vi "BuildCountertask.vi"(9 "Input Cluster":T2, 10 "Sample rate":dbl, 11 "Task cluster in":T1) -> (2 "CO.Pulse.Term":tag, 3 "Task cluster out":T1)   [LabVIEW 2018]
uses:
  Tasks_RT.ctl
  <vilib>/DAQmx/create/channels.llb/DAQmx Create Channel (CO-Pulse Generation-Frequency).vi
  <vilib>/DAQmx/configure/timing.llb/DAQmx Timing (Implicit).vi
  <vilib>/DAQmx/configure/trigger.llb/DAQmx Start Trigger (Digital Edge).vi
  <resource>/objmgr/daqmx.rc
panel:
  # "Tasks and errors"
  # "Tasks and errors"
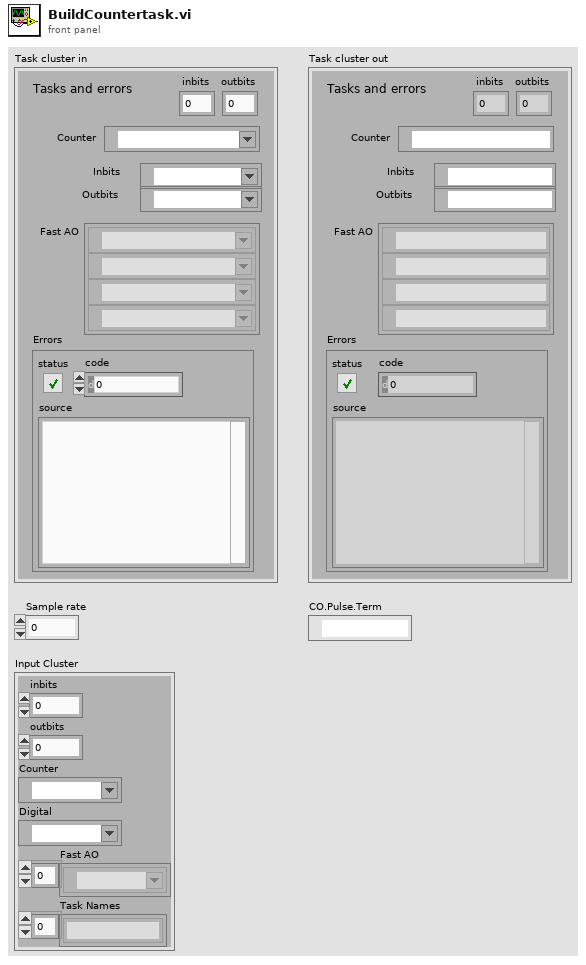
[diagram p1: front panel]
types:
  T1 = typedef "Tasks_RT.ctl" = cluster{"inbits":i32, "outbits":i32, "Counter":refnum<k21>, "Inbits":refnum<k21>, "Outbits":refnum<k21>, "Fast AO":refnum<k21>[], "Errors":errorcluster}
  T2 = cluster{"inbits":i32, "outbits":i32, "Counter":tag, "Digital":tag, "Fast AO":tag[], "Task Names":string[]}
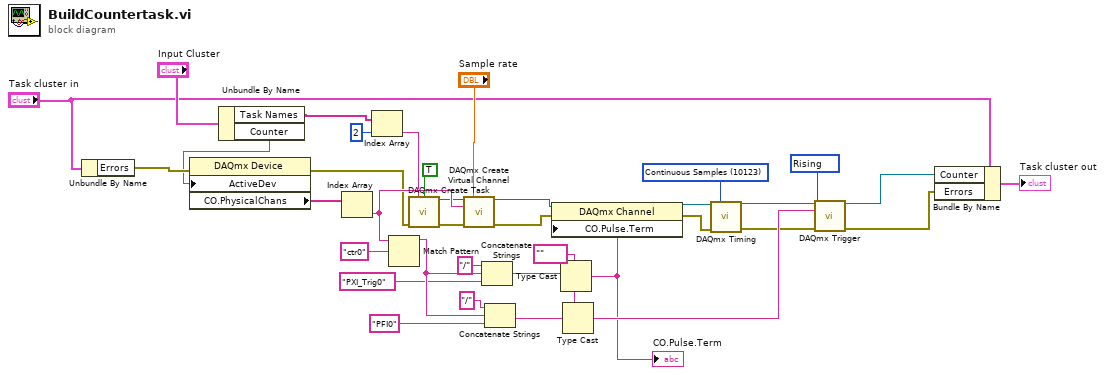
[diagram p0: block diagram]
diagram:
  w1 = 10280 items=["Rising"=10280, "Falling"=10171] ("edge")
  w22 = 10123 items=["Finite Samples"=10178, "Continuous Samples"=10123, "Hardware Timed Single Point"=12522] ("sample mode")
  w33 = tag "" ("CO.Pulse.Term")
  n1 = Unbundle By Name("Task cluster in") -> ("Errors"=w36:errorcluster)
  n2 = Unbundle By Name("Input Cluster") -> ("Task Names"=w13:string[], "Counter"=w4:tag)
  n3 = property class="DAQmx Device"(error in=w36, "ActiveDev"=w4) -> (error out=w15:errorcluster, "CO.PhysicalChans"=w14:tag[])  [unwired: 1 in, 1 out]
  n4 = Index Array(array=w14) -> (element=w16:tag)  [unwired: 1 in]
  n5 = Index Array(array=w13, index=2) -> (element=w12:string)
  n6 = Match Pattern(string=w16, regular expression="ctr0") -> (before substring=w29:string)  [unwired: 1 in, 3 out]
  n7 = call <vilib>:"DAQmx Create Task.vi"("new task name"=w12, "auto cleanup"=TRUE, "error in"=w15) -> ("task out"=w8:refnum<k21>, "error out"=w7:errorcluster)  [unwired: 11 in]
  n8 = call-poly <vilib>:"DAQmx Create Virtual Channel.vi"("task in"=w8, "frequency"="Sample rate", "counter"=w16, "error in"=w7) -> ("task out"=w5:refnum<k21>, "error out"=w6:errorcluster)  [unwired: 10 in]
  n9 = Concatenate Strings("/" ("string"), w29, "PXI_Trig0" ("string")) -> (w28:string)
  n10 = Concatenate Strings("/" ("string"), w29, "PFI0" ("string")) -> (w32:string)
  n11 = Type Cast(type=w33, x=w28) -> (*(type *) &x=w31:tag)
  "CO.Pulse.Term" <- w31
  n12 = property class="DAQmx Channel"(reference=w5, error in=w6, "CO.Pulse.Term"=w31) -> (reference out=w20:refnum<k21>, error out=w21:errorcluster)
  n13 = Type Cast(type=w33, x=w32) -> (*(type *) &x=w34:tag)
  n14 = call-poly <vilib>:"DAQmx Timing.vi"("task/channels in"=w20, "sample mode"=w22, "error in"=w21) -> ("task out"=w25:refnum<k21>, "error out"=w24:errorcluster)  [unwired: 11 in]
  n15 = call-poly <vilib>:"DAQmx Trigger.vi"("task/channels in"=w25, "source"=w34, "edge"=w1, "error in"=w24) -> ("task out"=w26:refnum<k21>, "error out"=w35:errorcluster)  [unwired: 10 in]
  n16 = Bundle By Name(cluster="Task cluster in", "Counter"=w26, "Errors"=w35) -> (→"Task cluster out":T1)
